vi "Write Setup Camera.vi"(8 "error in (no error)":errorcluster, 10 "RED Channel Settings":T1={"Cooler ON/OFF"=0, "Set temperature"=20.0, "Shutter Mode "=2, "Shutter TTL"=0, "Time to open (ms)"=50.0, "Time to close (ms)"=50.0, "Pre-amplifier gain"=1, "Vertical clock\n  voltage amplitude"=0, "Vertical Shift Speed"=0, "Readout Rate "=0, "Trigger "=0, "Conventional/EM"=1, "Read Mode "=4, "Acquisition Mode "=1, "Exposure Time (s) "=0.0, "Initial Line"=1, "Initial Column"=1, "Final Line"=1, "Final Column"=1, "Horizontal binning"=1, "Vertical binning "=1, "FITS Format"=0, "Image Format"="", "Tiff Position "=1, "Tiff Type"=0, "Image Path"=""} {"Tiff Type" items=["8-bit", "16-bit", "Color"]; "FITS Format" items=["Unsigned 16", "Unsigned 32", "Signed 16", "Signed 32", "Float"]; "Exposure Time (s)" format="%.2f"; "Acquisition Mode" items=["RESERVED", "Single Scan", "Accumulate", "Kinetics", "Fast Kinetics", "Run Til Abort", "RESERVED", "RESERVED", "RESERVED", "RESERVED", "Time Delayed Integration"]; "Read Mode" items=["Full Vertical Binning", "Multi-Track", "Random-Track", "Single-Track", "Image"]; "Conventional/EM" items=["EM Gain", "Conventional"]; "Trigger" items=["Internal", "External", "N/A", "N/A", "N/A", "N/A", "External Start", "External Exposure (bulb)", "N/A", "External FVB EM", "Software", "N/A", "External Charge Shifting"]; "Shutter TTL" items=["TTL Low", "TTL High"]; "Shutter Mode" items=["Fully Auto", "OPEN", "CLOSED"]; "Set temperature" min=-80.0 max=20.0; "Cooler ON/OFF" items=["Cooler OFF", "Cooler ON"]}, 11 "Construct String Setup Cam in":refnum<class "Construct String Setup Cam.lvclass">) -> (0 "error out":errorcluster, 3 "Construct String Setup Cam out":refnum<class "Construct String Setup Cam.lvclass">)   [LabVIEW 2018, in "Construct String Setup Cam.lvclass"]
doc: "Este VI recebe um cluster contendo a configuração da câmera, escrevendo essas informações na classe."
uses:
  Construct String Setup Cam.lvclass
  Construct String Setup Cam.lvclass/Construct String Setup Cam.ctl
panel:
  # "Set Shutter Configuration"
  # "Timings"
  # "Vertical pixel shift"
  # "(TTL level required to open \nyour external shutter)"
  # "Time to open/close shutter"
  # "Horizontal pixel shift"
  # "Temperature"
  # "Electron Multiplier (EM) Gain"
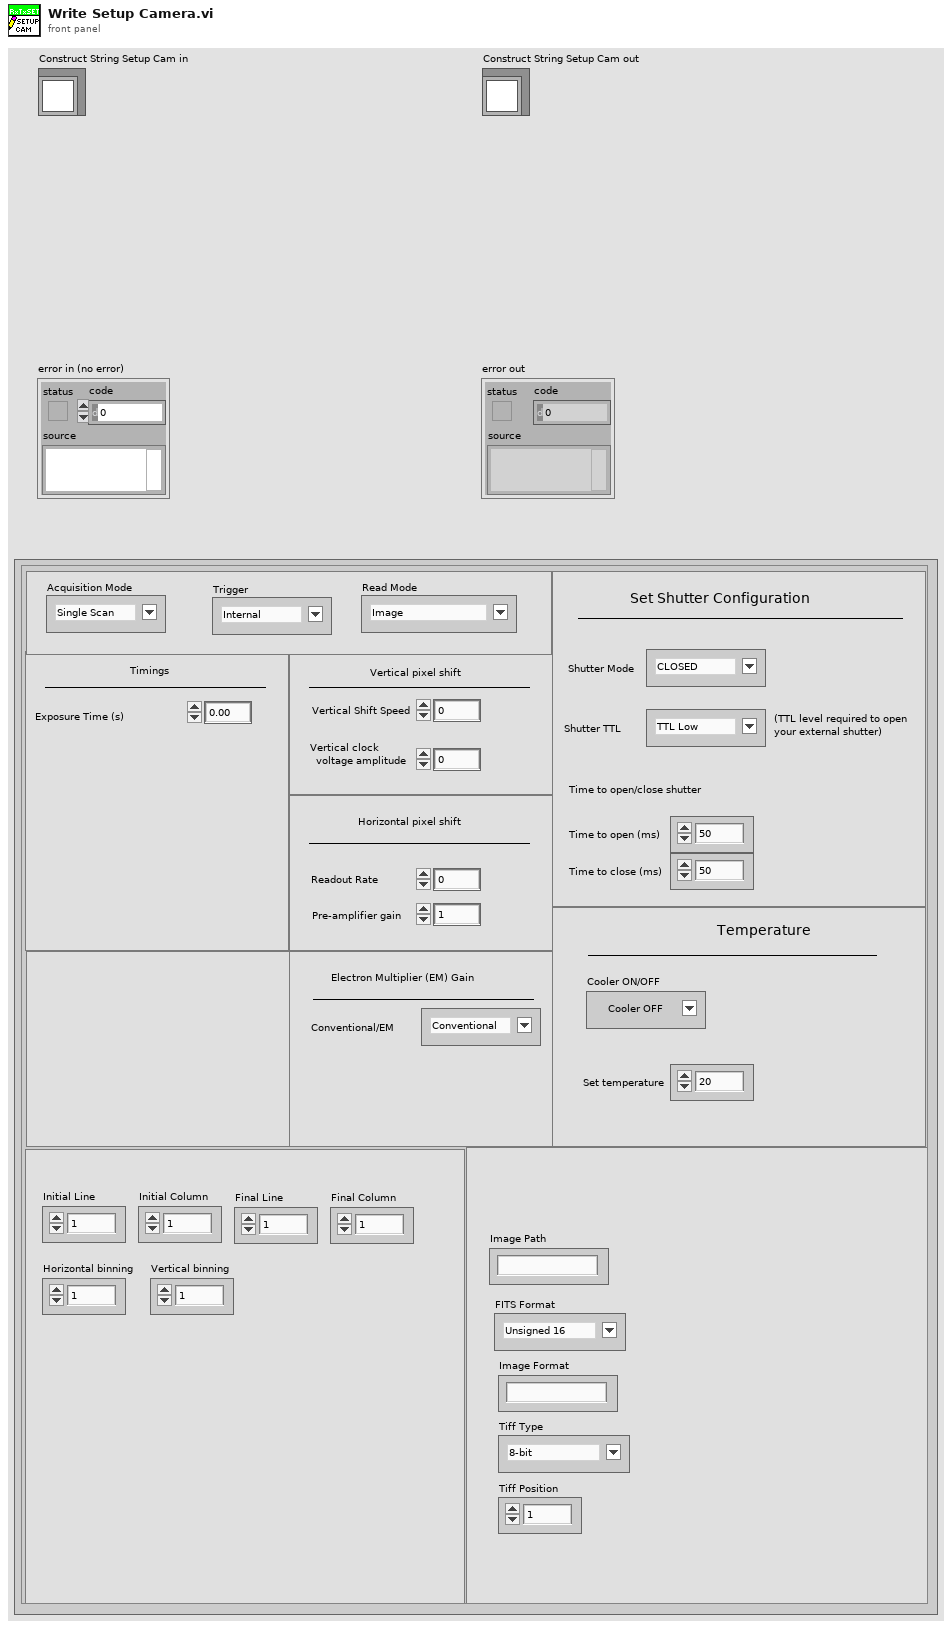
[diagram p1: front panel]
types:
  T1 = cluster{"Cooler ON/OFF":u16, "Set temperature":dbl, "Shutter Mode ":u16, "Shutter TTL":u16, "Time to open (ms)":dbl, "Time to close (ms)":dbl, "Pre-amplifier gain":i32, "Vertical clock\n  voltage amplitude":i32, "Vertical Shift Speed":i32, "Readout Rate ":i32, "Trigger ":u16, "Conventional/EM":i32, "Read Mode ":u16, "Acquisition Mode ":u16, "Exposure Time (s) ":sgl, "Initial Line":i32, "Initial Column":i32, "Final Line":i32, "Final Column":i32, "Horizontal binning":i32, "Vertical binning ":i32, "FITS Format":u16, "Image Format":string, "Tiff Position ":u16, "Tiff Type":u16, "Image Path":string}
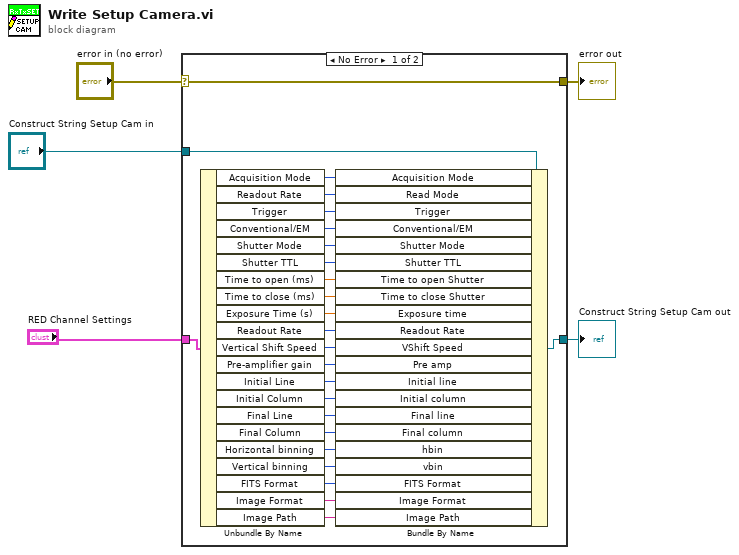
[diagram p0: block diagram]
diagram:
  n1 = case shown="No Error" "error in (no error)" {
    selector: "error in (no error)" -> [w30 w31]
    tunnel: [w30 w31] -> w4
    tunnel: [w28 w32] -> w2
    tunnel: "Construct String Setup Cam in" -> [w29 w32]
    tunnel: "RED Channel Settings" -> [w27 _]
    frame No Error {
      n2 = Unbundle By Name(w27) -> ("Acquisition Mode"=w26:u16, "Readout Rate"=w25:i32, "Trigger"=w24:u16, "Conventional/EM"=w23:i32, "Shutter Mode"=w22:u16, "Shutter TTL"=w21:u16, "Time to open (ms)"=w20:dbl, "Time to close (ms)"=w19:dbl, "Exposure Time (s)"=w18:sgl, "Readout Rate"=w17:i32, "Vertical Shift Speed"=w16:i32, "Pre-amplifier gain"=w15:i32, "Initial Line"=w14:i32, "Initial Column"=w13:i32, "Final Line"=w12:i32, "Final Column"=w11:i32, "Horizontal binning"=w10:i32, "Vertical binning"=w9:i32, "FITS Format"=w8:u16, "Image Format"=w7:string, "Image Path"=w6:string)
      n3 = Bundle By Name(cluster=w29, "Acquisition Mode"=w26, "Read Mode"=w25, "Trigger"=w24, "Conventional/EM"=w23, "Shutter Mode"=w22, "Shutter TTL"=w21, "Time to open Shutter"=w20, "Time to close Shutter"=w19, "Exposure time"=w18, "Readout Rate"=w17, "VShift Speed"=w16, "Pre amp"=w15, "Initial line"=w14, "Initial column"=w13, "Final line"=w12, "Final column"=w11, "hbin"=w10, "vbin"=w9, "FITS Format"=w8, "Image Format"=w7, "Image Path"=w6) -> (w28:refnum<class "Construct String Setup Cam.lvclass">)
    }
    frame Error {
    }
  }
  "error out" <- w4
  "Construct String Setup Cam out" <- w2
